vi "Set Image.vi"(8 "error in":errorcluster, 10 "Image":string, 11 "Cell in":refnum<class "Cell.lvclass">) -> (0 "error out":errorcluster, 3 "Cell out":refnum<class "Cell.lvclass">)   [LabVIEW 2023, in "SourceGrid.lvlib" / "Cell.lvclass"]
doc: "Sets Image from path"
uses:
  Cell.lvclass
  Cell.lvclass/Cell.ctl
  System.Drawing
  D:/git/Sourcegrid-LabVIEW/dll/SourceGrid.dll
  dll/SourceGrid.dll
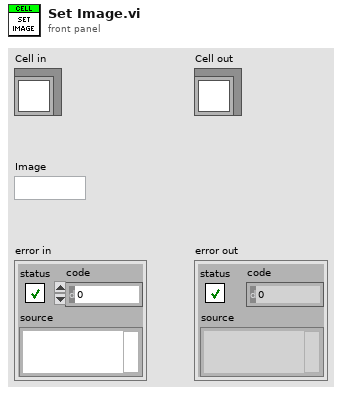
[diagram p1: front panel]
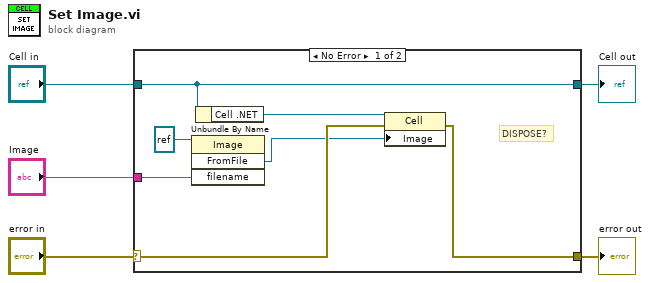
[diagram p0: block diagram]
diagram:
  n1 = case shown="No Error" "error in" {
    selector: "error in" -> [w11 w13]
    tunnel: [w10 w13] -> w4
    tunnel: [w8 w14] -> w2
    tunnel: "Cell in" -> [w8 w14]
    tunnel: "Image" -> [w7 _]
    frame No Error {
      # "DISPOSE?"
      n2 = invoke class="Image" method="FromFile"(reference=refnum<k24> refnum ("Image"), "filename"=w7) -> ("FromFile"=w6:refnum<k24>)  [unwired: 2 in, 3 out]
      n3 = Unbundle By Name(w8) -> ("Cell .NET"=w12:refnum<k24>)
      n4 = property class="Cell"(reference=w12, error in=w11, "Image"=w6) -> (error out=w10:errorcluster)  [unwired: 1 out]
    }
    frame Error {
    }
  }
  "error out" <- w4
  "Cell out" <- w2
